vi "Set Output FIFOs.vi"(10 "Output FIFOs":refnum<k33>, 11 "Output Process in":refnum<class "Sine Process.lvclass">) -> (3 "Output Process out":refnum<class "Sine Process.lvclass">)   [LabVIEW 2019, in "TimingDRV Engine.lvlib" / "Sine Process.lvclass"]
uses:
  Sine Process.lvclass
  Sine Process.lvclass/Sine Process.ctl
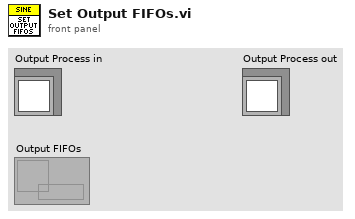
[diagram p1: front panel]
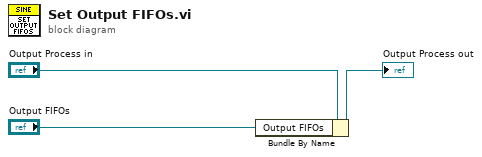
[diagram p0: block diagram]
diagram:
  n1 = Bundle By Name(cluster="Output Process in", "Output FIFOs"="Output FIFOs") -> (→"Output Process out":refnum<class "Sine Process.lvclass">)
